vi "WFDC Get Current XY Drift.vi"(0 "Center Ref Image":T1, 2 "hBox":i32, 7 "Current Image":u16[][](array[numeric]), 11 "Error In":errorcluster) -> (4 "Drift (px)":dbl[](array[numeric]), 8 "Corr Array":dbl[][](array[numeric]), 15 "Error Out":errorcluster)   [LabVIEW 2020]
uses:
  <vilib>/vision/Image Controls.llb/IMAQ Image.ctl
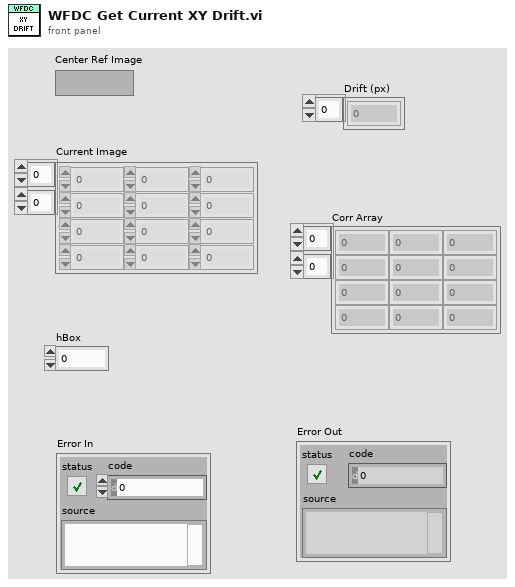
[diagram p1: front panel]
types:
  T1 = typedef "IMAQ Image.ctl" = refnum<image>
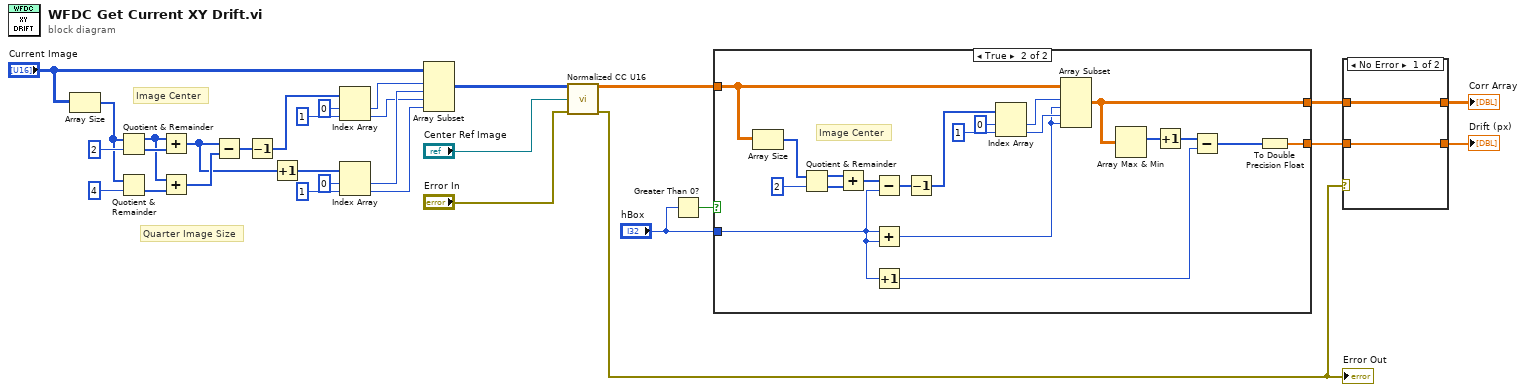
[diagram p0: block diagram]
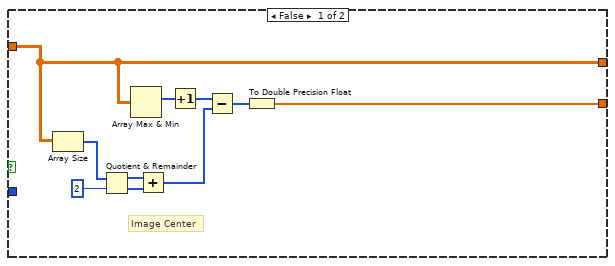
[diagram p2: hidden frame]
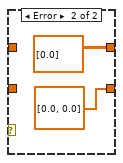
[diagram p3: hidden frame]
diagram:
  # "Quarter Image Size"
  # "Image Center"
  n1 = Array Size(array="Current Image") -> (size(s)=w26:i32[])
  n2 = Quotient & Remainder(x=w26, y=2) -> (x-y*floor(x/y)=w27:i32[], floor(x/y)=w29:i32[])
  n3 = Quotient & Remainder(x=w26, y=4) -> (floor(x/y)=w28:i32[])  [unwired: 1 out]
  n4 = Add(x=w27, y=w29) -> (x+y=w17:i32[])
  n5 = Add(x=w27, y=w28) -> (x+y=w24:i32[])
  n6 = Subtract(x=w17, y=w24) -> (x-y=w23:i32[])
  n7 = Decrement(x=w23) -> (x-1=w22:i32[])
  n8 = Increment(x=w17) -> (x+1=w6:i32[])
  n9 = Index Array(array=w22, index #1=0 ("index"), index #2=1 ("index")) -> (element #1=w5:i32, element #2=w4:i32)
  n10 = Index Array(array=w6, index #1=0 ("index"), index #2=1 ("index")) -> (element #1=w16:i32, element #2=w15:i32)
  n11 = Array Subset(array="Current Image", index (row)=w5, length (row)=w16, index (col)=w4, length (col)=w15) -> (w8:u16[][])
  n12 = call "Normalized CC U16.vi"("Template U16"=w8, "A U16"="Center Ref Image", "Error In"="Error In") -> ("normxcorr2"=w13:dbl[][], "Error Out"=w11:errorcluster)  [unwired: 10 in, 1 out]
  "Error Out" <- w11
  n13 = Greater Than 0?(x="hBox") -> (x > 0?=w9:bool)
  n14 = case shown="True" w9 {
    tunnel: w13 -> [w35 w54]
    tunnel: "hBox" -> [_ w49]
    tunnel: [w35 w44] -> w12
    tunnel: [w32 w42] -> w2
    frame False {
      # "Image Center"
      n15 = Array Size(array=w35) -> (size(s)=w38:i32[])
      n16 = Quotient & Remainder(x=w38, y=2) -> (x-y*floor(x/y)=w39:i32[], floor(x/y)=w40:i32[])
      n17 = Array Max & Min(array=w35) -> (max index (indices)=w37:i32[])  [unwired: 3 out]
      n18 = Add(x=w39, y=w40) -> (x+y=w34:i32[])
      n19 = Increment(x=w37) -> (x+1=w33:i32[])
      n20 = Subtract(x=w33, y=w34) -> (x-y=w36:i32[])
      n21 = To Double Precision Float(number=w36) -> (double precision float=w32:dbl[])
    }
    frame True {
      # "Image Center"
      n22 = Array Size(array=w54) -> (size(s)=w58:i32[])
      n23 = Quotient & Remainder(x=w58, y=2) -> (x-y*floor(x/y)=w59:i32[], floor(x/y)=w60:i32[])
      n24 = Add(x=w59, y=w60) -> (x+y=w57:i32[])
      n25 = Subtract(x=w57, y=w49) -> (x-y=w53:i32[])
      n26 = Add(x=w49, y=w49) -> (x+y=w51:i32)
      n27 = Increment(x=w49) -> (x+1=w47:i32)
      n28 = Decrement(x=w53) -> (x-1=w50:i32[])
      n29 = Index Array(array=w50, index #1=0 ("index"), index #2=1 ("index")) -> (element #1=w56:i32, element #2=w52:i32)
      n30 = Array Subset(array=w54, index (row)=w56, length (row)=w51, index (col)=w52, length (col)=w51) -> (w44:dbl[][])
      n31 = Array Max & Min(array=w44) -> (max index (indices)=w48:i32[])  [unwired: 3 out]
      n32 = Increment(x=w48) -> (x+1=w43:i32[])
      n33 = Subtract(x=w43, y=w47) -> (x-y=w45:i32[])
      n34 = To Double Precision Float(number=w45) -> (double precision float=w42:dbl[])
    }
  }
  n35 = case shown="No Error" w11 {
    tunnel: w12 -> [w63 _]
    tunnel: [w63 dbl[][] [[0.0]]] -> w3
    tunnel: w2 -> [w62 _]
    tunnel: [w62 dbl[] [0.0, 0.0]] -> w1
    frame No Error {
    }
    frame Error {
    }
  }
  "Corr Array" <- w3
  "Drift (px)" <- w1
